vi "Validate.vi"() -> ()   [LabVIEW 2021, in "Online_TRAC.lvclass"]
uses:
  Online_TRAC.lvclass
  Online_TRAC.lvclass/Online_TRAC.ctl
panel:
  out "TRAC Sine Sine":dbl
  out "Cosine":dbl(graph)
  out "Sine":dbl(graph)
  out "TRAC Sine Cosine":dbl
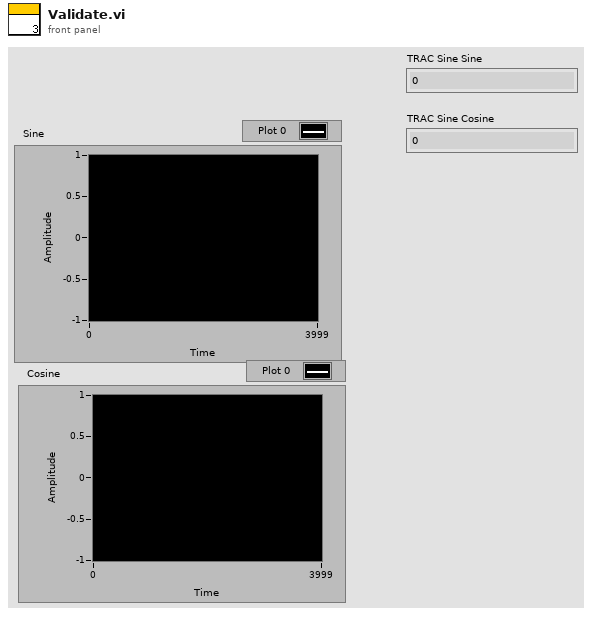
[diagram p1: front panel]
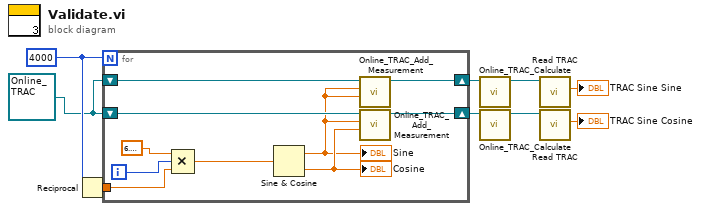
[diagram p0: block diagram]
diagram:
  w8 = 4000
  w4 = refnum<class "Online_TRAC.lvclass"> refnum ("Online_TRAC.lvclass")
  n1 = Reciprocal(x=w8) -> (1/x=w7:dbl)
  n2 = for {
    N: w8 -> [_]
    shift-right: [w18] -> w6
    shift-left: w4 -> [w19]
    tunnel: w7 -> [w17]
    shift-right: [w12] -> w2
    shift-left: w4 -> [w13]
    i -> [w16]
    n3 = Compound Arithmetic op=MULTIPLY(6.283185307179586, w16, w17) -> (w14:dbl)
    n4 = Sine & Cosine(0:w14) -> (1:w10:dbl, 2:w11:dbl)
    "Sine" <- w10
    "Cosine" <- w11
    n5 = call-dynamic "Online_TRAC_Add_Measurement.vi"("Estimate"=w10, "True"=w10, "Online_TRAC in"=w13) -> ("Online_TRAC out"=w12:refnum<class "Online_TRAC.lvclass">)  [unwired: 7 in, 1 out]
    n6 = call-dynamic "Online_TRAC_Add_Measurement.vi"("Estimate"=w11, "True"=w10, "Online_TRAC in"=w19) -> ("Online_TRAC out"=w18:refnum<class "Online_TRAC.lvclass">)  [unwired: 7 in, 1 out]
  }
  n7 = call "Online_TRAC_Calculate.vi"("Online_TRAC in"=w2) -> ("Online_TRAC out"=w3:refnum<class "Online_TRAC.lvclass">)  [unwired: 9 in, 1 out]
  n8 = call "Online_TRAC_Calculate.vi"("Online_TRAC in"=w6) -> ("Online_TRAC out"=w5:refnum<class "Online_TRAC.lvclass">)  [unwired: 9 in, 1 out]
  n9 = call "Read TRAC.vi"("Online_TRAC in"=w3) -> ("TRAC"=→"TRAC Sine Sine":dbl)  [unwired: 8 in, 2 out]
  n10 = call "Read TRAC.vi"("Online_TRAC in"=w5) -> ("TRAC"=→"TRAC Sine Cosine":dbl)  [unwired: 8 in, 2 out]
